vi "Define 2D Heat PDE IC (VIRef).vi"(0 "PDE in":refnum<class "NI_PDE.lvclass">, 1 "data":variant, 5 "Initial Condition":refnum<vi>, 11 "error in (no error)":errorcluster) -> (4 "PDE out":refnum<class "NI_PDE.lvclass">, 15 "error out":errorcluster)   [LabVIEW 2017, in "NI_PDE.lvlib"]
doc: "Defines the initial condition of a partial differential equation. You must manually select the polymorphic instance to use."
uses:
  <vilib>/gmath/NI_PDE.lvlib
  <vilib>/gmath/pde.llb/PDEClass/NI_PDE.lvclass
  <vilib>/gmath/pde.llb/ICClass/IC_2D_VIRef/NI_IC_2D_VIRef.lvclass
  e:/builds/penguin/labview/branches/2017/dev/dist/vi.lib/gmath/pde.llb/ICClass/NI_IC.lvclass
  <vilib>/gmath/pde.llb/PDEClass/PDE_Heat_2D/NI_PDE_Heat_2D.lvclass
  e:/builds/penguin/labview/branches/2017/dev/dist/vi.lib/gmath/pde.llb/PDEClass/NI_PDE.lvclass
  <vilib>/gmath/pde.llb/Common/PDE_IC Type.ctl
  <vilib>/gmath/pde.llb/ICClass/IC_2D_VIRef/IC Data.ctl
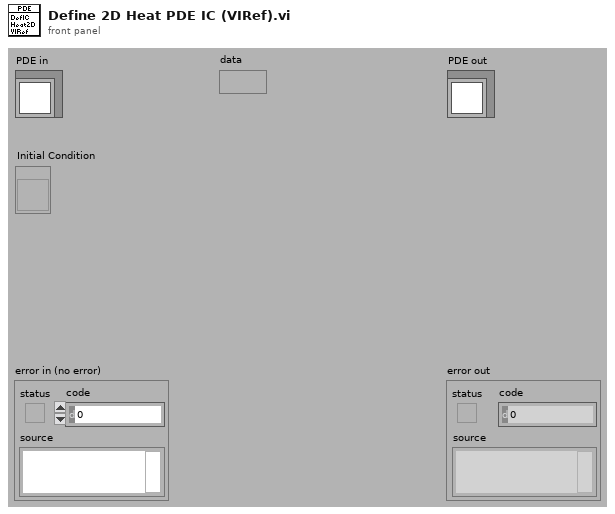
[diagram p1: front panel]
types:
  T1 = typedef "NI_PDE.lvlib/PDE_IC Type.ctl" = i32
  T2 = typedef "NI_PDE.lvlib/NI_IC_2D_VIRef.lvclass/IC Data.ctl" = cluster{"type":T1, "H":refnum<vi>, "data":variant}
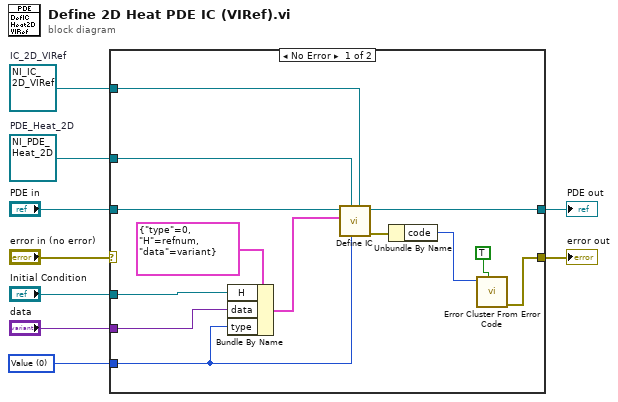
[diagram p0: block diagram]
diagram:
  w3 = T1 0 items=["Value", "Derivative"] ("type")
  w2 = refnum<class "NI_PDE_Heat_2D.lvclass"> refnum  # PDE_Heat_2D
  w1 = refnum<class "NI_IC_2D_VIRef.lvclass"> refnum  # IC_2D_VIRef
  n1 = case shown="No Error" "error in (no error)" {
    selector: "error in (no error)" -> [_ w24]
    tunnel: "PDE in" -> [w10 w23]
    tunnel: [w17 w23] -> w8
    tunnel: "data" -> [w14 _]
    tunnel: "Initial Condition" -> [w13 _]
    tunnel: [w20 w24] -> w5
    tunnel: w3 -> [w15 _]
    tunnel: w2 -> [w12 _]
    tunnel: w1 -> [w11 _]
    frame No Error {
      n2 = Bundle By Name(cluster=T2 {"type"=0, "H"=refnum, "data"=variant} ("IC data"), "H"=w13, "data"=w14, "type"=w15) -> (w19:T2)
      n3 = call <vilib>:"Define IC.vi"("target IC"=w11, "index"=w15, "target PDE"=w12, "IC"=w19, "PDE in"=w10) -> ("error out"=w16:errorcluster, "PDE out"=w17:refnum<class "NI_PDE.lvclass">)  [unwired: 2 in, 3 out]
      n4 = Unbundle By Name(w16) -> ("code"=w22:i32)
      n5 = call <vilib>:"Error Cluster From Error Code.vi"("show call chain? (False)"=TRUE, "error code (0)"=w22) -> ("error out"=w20:errorcluster)  [unwired: 1 in, 6 out]
    }
    frame Error {
    }
  }
  "PDE out" <- w8
  "error out" <- w5
